vi "SLSC Get Module Name from IP Address.vi"(5 "Password":string, 6 "connect timeout":dbl=50.0, 7 "Username":string="admin", 8 "Error In":errorcluster, 10 "Slot #":u32=6, 11 "Chassis IP Address":string="192.168.8.130") -> (0 "Error Out":errorcluster, 1 "SLSC Chassis Name":string, 3 "SLSC Module Name":string)   [LabVIEW 2017]
uses:
  <vilib>/nisyscfg/Close (System).vi
  <vilib>/SLSC/Initialize Session with Devices.vi
  <vilib>/SLSC/Initialize Session without Resources.vi
  <vilib>/SLSC/Close Session.vi
  <vilib>/SLSC/SLSC.lvlib
  <resource>/objmgr/slsc.rc
  <vilib>/nisyscfg/nisyscfg.lvlib
  <resource>/objmgr/nisysapi.rc
  SLSC CD Engine.lvlib
panel:
  out "concatenated string":string
  out "session out debug":string
  out "Dev.SlotNum":u32
  out "Module Found?":bool
  out "Host Name":string
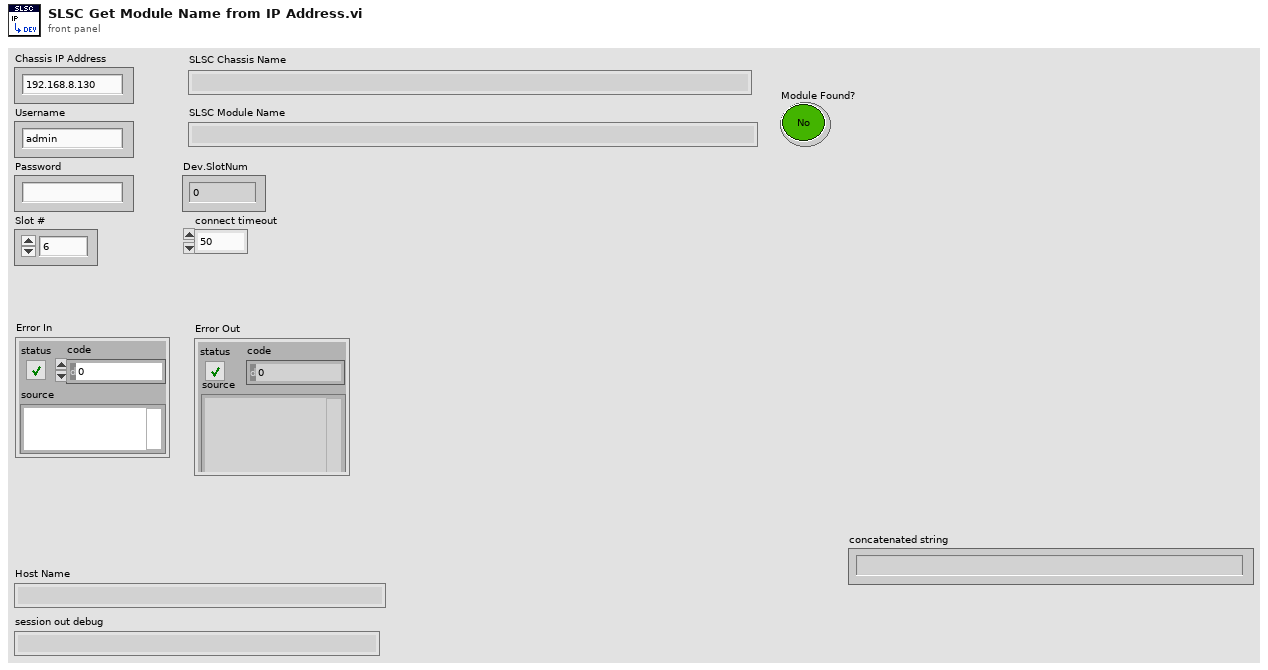
[diagram p1: front panel]
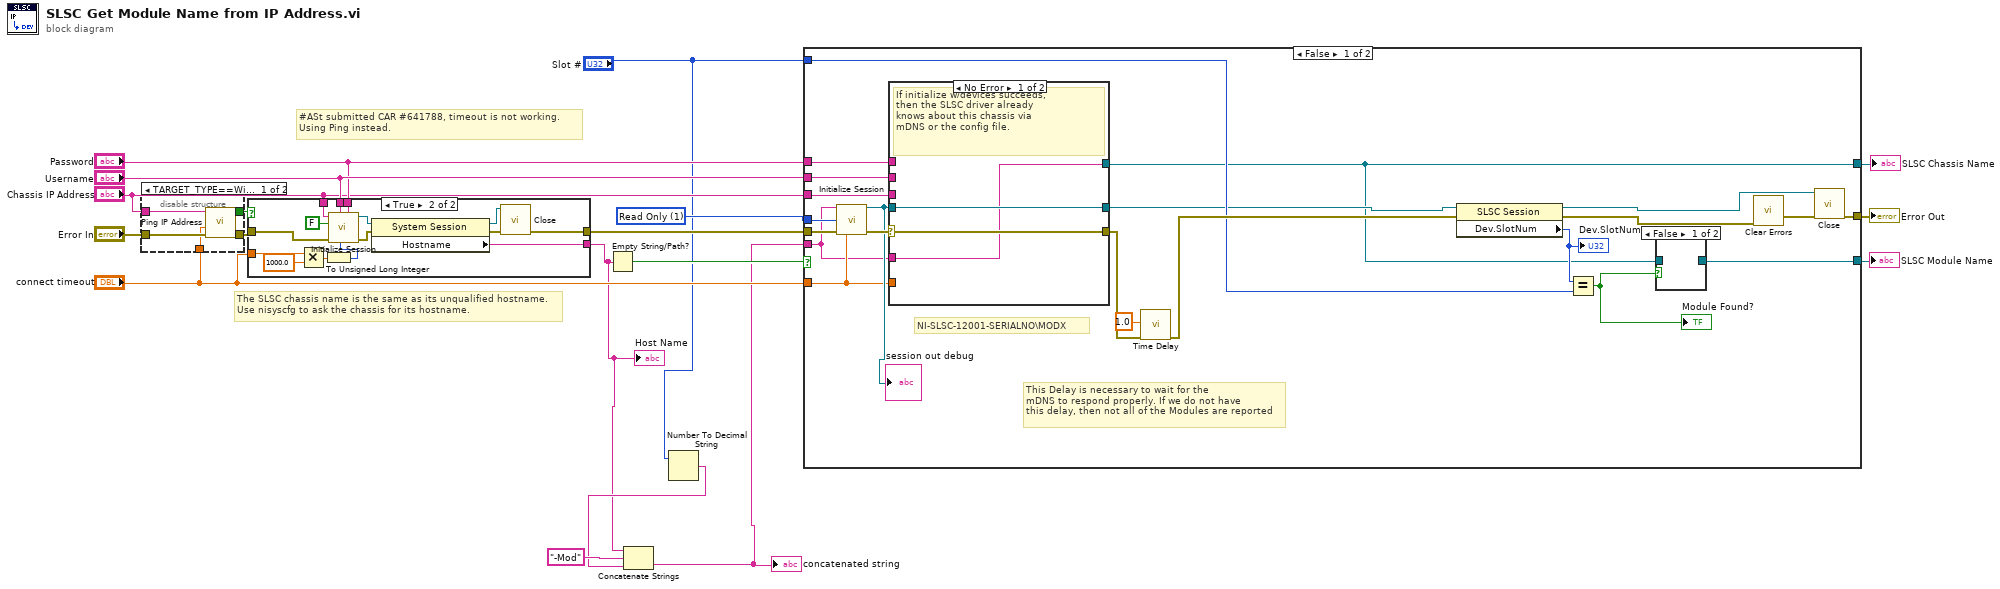
[diagram p0: block diagram]
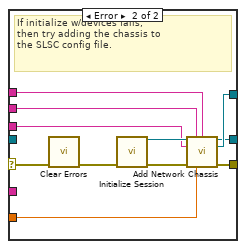
[diagram p3: hidden frame]
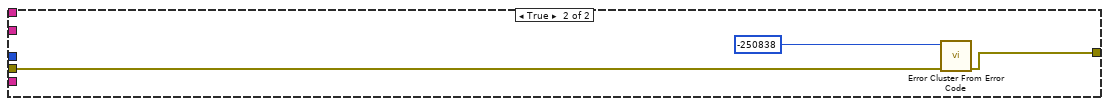
[diagram p4: hidden frame]
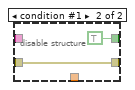
[diagram p5: hidden frame]
diagram:
  w18 = 1 items=["None"=0, "Read Only"=1, "Read/Write"=3] ("reservation access (Read/Write)")
  # "#ASt submitted CAR #641788, timeout is not working.\nUsing Ping instead."
  # "The SLSC chassis name is the same as its unqualified hostname.\nUse nisyscfg to ask the chassis for its hostname."
  n1 = disable-structure shown="TARGET_TYPE==Windows" {
    disable-tunnel: "Chassis IP Address" -> [w23 _]
    disable-tunnel: [w22 TRUE ("response?")] -> w13
    disable-tunnel: "Error In" -> [w21 w25]
    disable-tunnel: [w20 w25] -> w11
    disable-tunnel: "connect timeout" -> [w19 _]
    frame condition #0 (active) {
      n2 = call "Ping IP Address.vi"("error in"=w21, "timeout (500 ms)"=w19, "host"=w23) -> ("error out"=w20:errorcluster, "response?"=w22:bool)  [unwired: 6 in, 1 out]
    }
    frame condition #1 {
    }
  }
  n3 = case shown="True" w13 {
    tunnel: [w26 w37] -> w9
    tunnel: w11 -> [w26 w33]
    tunnel: "Username" -> [_ w32]
    tunnel: "Password" -> [_ w31]
    tunnel: "connect timeout" -> [_ w30]
    tunnel: [_ w28] -> w2
    tunnel: "Chassis IP Address" -> [_ w27]
    frame False {
    }
    frame True {
      n4 = Multiply(x=w30, y=1000.0) -> (x*y=w35:dbl)
      n5 = To Unsigned Long Integer(number=w35) -> (unsigned 32bit integer=w34:u32)
      n6 = call <vilib>:"Initialize Session.vi"("Password"=w31, "Connect Timeout (4000 ms)"=w34, "User Name"=w32, "error in (no error)"=w33, "Force Property Refresh (T)"=FALSE, "Target (localhost)"=w27) -> ("error out"=w40:errorcluster, "Session out"=w41:refnum<k21>)  [unwired: 4 in]
      n7 = property class="System Session"(reference=w41, error in=w40) -> (reference out=w38:refnum<k21>, error out=w39:errorcluster, "Hostname"=w28:string)
      n8 = call-poly <vilib>:"Close.vi"("error in (no error)"=w39, "Session in"=w38) -> ("error out"=w37:errorcluster)  [unwired: 9 in]
    }
  }
  "Host Name" <- w2
  n9 = Empty String/Path?(string/path=w2) -> (empty?=w15:bool)
  n10 = Number To Decimal String(number="Slot #") -> (decimal integer string=w6:string)  [unwired: 1 in]
  n11 = Concatenate Strings(w2, "-Mod" ("string"), w6) -> (w1:string)
  "concatenated string" <- w1
  n12 = case shown="False" w15 {
    tunnel: [w51 w81] -> w5
    tunnel: w9 -> [w62 w79]
    tunnel: w18 -> [w61 _]
    tunnel: "Chassis IP Address" -> [w58 _]
    tunnel: "Username" -> [w57 _]
    tunnel: "Password" -> [w56 _]
    tunnel: [w43 _] -> w4
    tunnel: "connect timeout" -> [w54 _]
    tunnel: [w53 _] -> w3
    tunnel: w1 -> [w52 _]
    tunnel: "Slot #" -> [w47 _]
    frame False {
      # "This Delay is necessary to wait for the \nmDNS to respond properly. If we do not have\nthis delay, then not all of the Modules are reported"
      # "NI-SLSC-12001-SERIALNO\\MODX"
      n13 = call-poly <vilib>:"Initialize Session.vi"("devices"=w52, "reservation access (Read/Write)"=w61, "error in (no error)"=w62, "connect timeout (60 sec)"=w54) -> ("session out"=w59:refnum<k21>, "error out"=w60:errorcluster)  [unwired: 10 in]
      "session out debug" <- w59
      n14 = case shown="No Error" w60 {
        selector: w60 -> [w67 w78]
        tunnel: [w67 w70] -> w50
        tunnel: [w66 w71] -> w44
        tunnel: w59 -> [w66 _]
        tunnel: w58 -> [_ w76]
        tunnel: w57 -> [_ w74]
        tunnel: w56 -> [_ w73]
        tunnel: [w65 w72] -> w43
        tunnel: w52 -> [w65 _]
        tunnel: w54 -> [_ w68]
        frame No Error {
          # "If initialize w/devices succeeds,\nthen the SLSC driver already\nknows about this chassis via\nmDNS or the config file."
        }
        frame Error {
          # "If initialize w/devices fails,\nthen try adding the chassis to\nthe SLSC config file."
          n15 = call <vilib>:"Clear Errors.vi"("error in (no error)"=w78) -> ("error out"=w69:errorcluster)  [unwired: 5 in, 1 out]
          n16 = call-poly <vilib>:"Initialize Session.vi"("error in (no error)"=w69) -> ("session out"=w77:refnum<k21>, "error out"=w75:errorcluster)  [unwired: 13 in]
          n17 = call <vilib>:"Add Network Chassis.vi"("session in"=w77, "username"=w74, "password"=w73, "chassis IP address/hostname"=w76, "error in (no error)"=w75, "connect timeout (60 sec)"=w68) -> ("session out"=w71:refnum<k21>, "chassis out"=w72:refnum<k21>, "error out"=w70:errorcluster)  [unwired: 7 in]
        }
      }
      n18 = call "Time Delay"("error in (no error)"=w50, "Delay Time (s)"=1.0) -> ("error out"=w49:errorcluster)  [unwired: 9 in]
      n19 = property class="SLSC Session"(reference=w44, error in=w49) -> (reference out=w63:refnum<k21>, error out=w55:errorcluster, "Dev.SlotNum"=w45:u32)
      "Dev.SlotNum" <- w45
      n20 = Equal?(x=w45, y=w47) -> (x = y?=w46:bool)
      "Module Found?" <- w46
      n21 = case shown="False" w46 {
        tunnel: w43 -> [_ w64]
        tunnel: [_ w64] -> w53
        frame False {
        }
        frame True {
        }
      }
      n22 = call <vilib>:"Clear Errors.vi"("error in (no error)"=w55) -> ("error out"=w42:errorcluster)  [unwired: 5 in, 1 out]
      n23 = call-poly <vilib>:"Close.vi"("session in"=w63, "error in (no error)"=w42) -> ("error out"=w51:errorcluster)  [unwired: 13 in]
    }
    frame True {
      n24 = call <vilib>:"Error Cluster From Error Code.vi"("error in (no error)"=w79, "error code (0)"=-250838 ("code")) -> ("error out"=w81:errorcluster)  [unwired: 7 in]
    }
  }
  "SLSC Chassis Name" <- w4
  "Error Out" <- w5
  "SLSC Module Name" <- w3
